vi "WaveSineGen.vi"(9 "Stop":refnum<vi>, 10 "Wave out":refnum<vi>, 11 "Frequncy":refnum<vi>) -> ()   [LabVIEW 2016]
panel:
  out "Waveform Chart":dbl(graph)
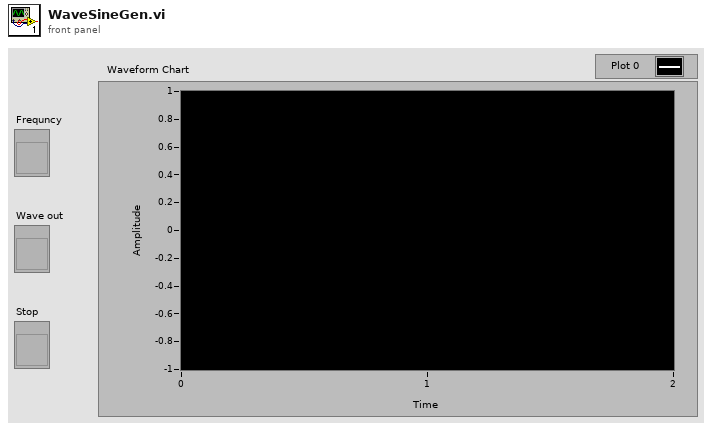
[diagram p1: front panel]
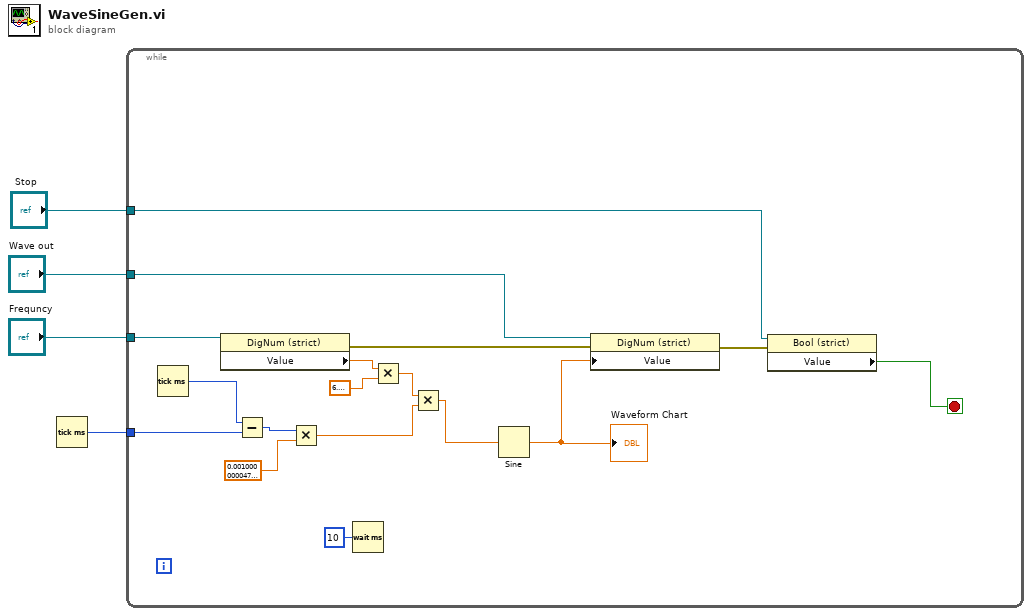
[diagram p0: block diagram]
diagram:
  n1 = Tick Count (ms)() -> (millisecond timer value=w1:u32)
  n2 = while {
    tunnel: "Frequncy" -> [w21]
    tunnel: "Wave out" -> [w19]
    tunnel: "Stop" -> [w16]
    tunnel: w1 -> [w11]
    stop <- w15 stop-if-true
    n3 = Tick Count (ms)() -> (millisecond timer value=w12:u32)
    n4 = property class="DigNum (strict)"(reference=w21) -> (error out=w18:errorcluster, "Value"=w14:dbl)  [unwired: 1 in, 1 out]
    n5 = Subtract(x=w12, y=w11) -> (x-y=w7:u32)
    n6 = Multiply(x=w7, y=sgl 0.001) -> (x*y=w5:sgl)
    n7 = Wait (ms)(milliseconds to wait=u32 10) -> ()  [unwired: 1 out]
    n8 = Multiply(x=w14, y=6.283185307179586) -> (x*y=w10:dbl)
    n9 = Multiply(x=w10, y=w5) -> (x*y=w9:dbl)
    n10 = Sine(x=w9) -> (sin(x)=w20:dbl)
    "Waveform Chart" <- w20
    n11 = property class="DigNum (strict)"(reference=w19, error in=w18, "Value"=w20) -> (error out=w17:errorcluster)  [unwired: 1 out]
    n12 = property class="Bool (strict)"(reference=w16, error in=w17) -> ("Value"=w15:bool)  [unwired: 2 out]
  }
